vi "RT_Refresh_Connections.vi"(8 "Error In":errorcluster, 11 "connection manager ref in":T1) -> (0 "Error Out":errorcluster, 3 "connection manager ref out":T1)   [LabVIEW 2018]
uses:
  <vilib>/NI/STM/Connection Manager/TCP/Advanced/TCP Connection Manager Reference.ctl
  <vilib>/NI/STM/Connection Manager/TCP/Advanced/TCP Connection Manager State Variables.ctl
  <vilib>/NI/STM/TCP/TCP Connection Info.ctl
  <vilib>/NI/STM/SubVIs/MetaDataElement.ctl
  <vilib>/NI/STM/Connection Manager/TCP/TCP Connection Properties.ctl
  <vilib>/NI/STM/Connection Manager/TCP/TCP Connection Method.ctl
  RT_Counter_FGV_States.ctl
  <vilib>/NI/STM/SubVIs/Generate STM Error.vi
  <vilib>/NI/STM/NI STM.lvlib
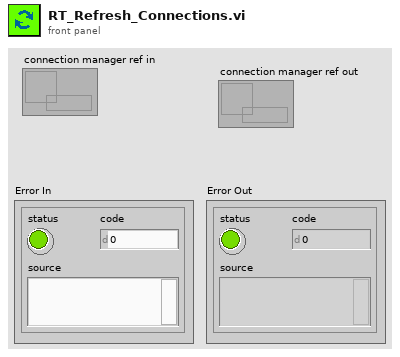
[diagram p1: front panel]
types:
  T1 = typedef "NI STM.lvlib/TCP Connection Manager Reference.ctl" = refnum<data-value>
  T2 = typedef "NI STM.lvlib/TCP Connection Method.ctl" = enum16{"Initialize", "Add Connection", "Set Properties", "Get Connection(s)", "Remove Connection", "Remove All Connections", "Get Connection Count"}
  T3 = typedef "RT_Counter_FGV_States.ctl" = enum16{"Init", "Increase", "Decrease", "Get"}
  T4 = typedef "NI STM.lvlib/TCP Connection Info.ctl" = cluster{"connection ID":refnum<k5>, "meta data":T5[]}
  T5 = typedef "NI STM.lvlib/MetaDataElement.ctl" = string
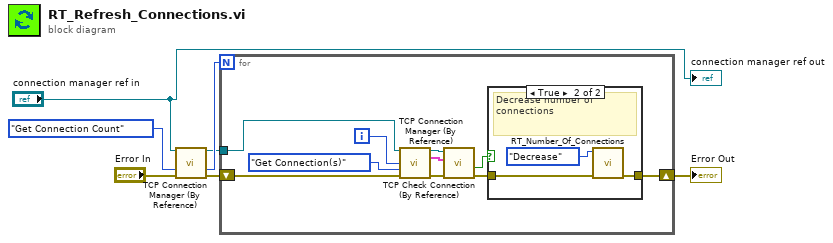
[diagram p0: block diagram]
diagram:
  n1 = call <vilib>:"TCP Connection Manager (By Reference).vi"("connection manager ref in"="connection manager ref in", "method"=TCP_Connection_Method."Get Connection Count", "error in"="Error In") -> ("connection manager ref out"=w5:T1, "number of connections"=w6:i32, "error out"=w4:errorcluster)  [unwired: 6 in, 4 out]
  n2 = for {
    N: w6 -> [_]
    tunnel: w5 -> [w17]
    shift-right: [w8] -> w2
    shift-left: w4 -> [w16]
    i -> [w15]
    n3 = call <vilib>:"TCP Connection Manager (By Reference).vi"("connection manager ref in"=w17, "index"=w15, "method"=TCP_Connection_Method."Get Connection(s)", "error in"=w16) -> ("connection manager ref out"=w11:T1, "connection out"=w12:T4, "error out"=w13:errorcluster)  [unwired: 5 in, 4 out]
    n4 = call <vilib>:"TCP Check Connection (By Reference).vi"("error in"=w13, "connection in"=w12, "connection manager ref in"=w11) -> ("error out"=w9:errorcluster, "disconnected?"=w10:bool)  [unwired: 4 in, 3 out]
    n5 = case shown="True" w10 {
      tunnel: w9 -> [w18 w20]
      tunnel: [w18 w19] -> w8
      frame False {
      }
      frame True {
        # "Decrease number of connections"
        n6 = call "RT_Number_Of_Connections.vi"("Error In"=w20, "Counter_FGV_States"=RT_Counter_FGV_States."Decrease") -> ("Error Out"=w19:errorcluster)  [unwired: 8 in, 1 out]
      }
    }
  }
  "Error Out" <- w2
  "connection manager ref out" <- "connection manager ref in"
